vi "Initialisieren.vi"(5 "YAchsen%Max":dbl=1.2, 6 "MFC Cluster Array":refnum<vi>[](array[refnum]), 7 "TestKonfig (Eingang)":T1 {"TestKonfig Interferent"."Gasflasche MFC3" items=["----"=10000, "IAG NH3 3000"=0, "IAG NH3 200"=1, "IAG NH3 2000"=2, "IAG MG"=3, "IAG O2"=4]; "TestKonfig Interferent"."Gasflasche MFC2" items=["----"=10000, "IAG NH3 3000"=0, "IAG NH3 200"=1, "IAG NH3 2000"=2, "IAG MG"=3, "IAG O2"=4]; "TestKonfig Interferent"."Eingangs Konzentration MFC1" min=0.0; "TestKonfig Interferent"."Ausgangs Konzentration MFC1" min=0.0; "TestKonfig Interferent"."MFC2" items=["MFC 2", "MFC 3", "MFC 4", "MFC 5"]; "TestKonfig Interferent"."MFC3" items=["MFC 2", "MFC 3", "MFC 4", "MFC 5"]; "TestKonfig Interferent"."Ausgangs Konzentration MFC3" min=0.0; "TestKonfig Interferent"."Eingangs Konzentration MFC3" min=0.0; "TestKonfig Interferent"."Ausgangs Konzentration MFC2" min=0.0; "TestKonfig Interferent"."Eingangs Konzentration MFC2" min=0.0; "TestKonfig H2O"."HovaCAL Temperature" format="%.2f"; "TestKonfig H2O"."HovaCAL Flow Input Cluster"."HovaCAL Flow Input Cluster" format="%.2f"; "TestKonfig H2O"."Eingangs Konzentration:" min=0.0; "TestKonfig H2O"."zusätzliche Zeitdauer Erster Punkt" min=30 step=1 format="%#_5g"; "TestKonfig H2O"."Zeitdauer Stufen" format="%#_5g"; "TestKonfig H2O"."Max Fehler" format="%#_5g"; "TestKonfig H2O"."Anzahl Stufen" format="%#_5g"; "TestKonfig H2O"."Modus" items=["Messen", "CG zu Entnahmestelle"]}, 8 "Fehler (Eingang)":errorcluster, 9 "Strings Array in":refnum<vi>[](array[refnum]), 10 "Ergebnis  Array in":refnum<vi>[](array[refnum]), 11 "Signalverlaufsdiagramm (Eingang)":refnum<vi>[](array[refnum])) -> (0 "Fehler (Ausgang)":errorcluster, 1 "Strings Array out":refnum<vi>[](array[refnum]), 2 "Ergenis Arry out":refnum<vi>[](array[refnum]), 3 "Signalverlaufsdiagramm (Ausgang)":refnum<vi>[](array[refnum]))   [LabVIEW 2020, in "EPA 1065.lvlib" / "HovaCAL Interference verificaton.lvlib"]
uses:
  HovaCAL Interference verificaton.lvlib
  TestKonfig.ctl
  TestKonfig H2O.ctl
  Modus.ctl
  Linearisierung V2/SpanEinstellungen/Einheit.ctl
  Linearisierung V2/Gasteiler/Stufen Tabelle 10 Stufen.ctl
  Linearisierung V2/Gasteiler/HovaCAL_Interface/Controls/Flow Einstellung.ctl
  Linearisierung V2/Gasteiler/HovaCAL_Interface/Controls/Temp Sollwerte Anzeige.ctl
  TestKonfig Interferents.ctl
  MFCAuswahl.ctl
  Seiten/System Einstellungen V2/Gasflasche Auswahl.ctl
  Linearisierung V2/SpanEinstellungen/SpanEinstellungen.lvlib
  Linearisierung V2/Gasteiler/HovaCAL_Interface/Controls/Controls.lvlib
  Seiten/System Einstellungen V2/System Einstellungen V2.lvlib
  Linearisierung V2/Gasteiler/Gasteiler.lvlib
panel:
  # "sec"
  # "%"
  # "sec"
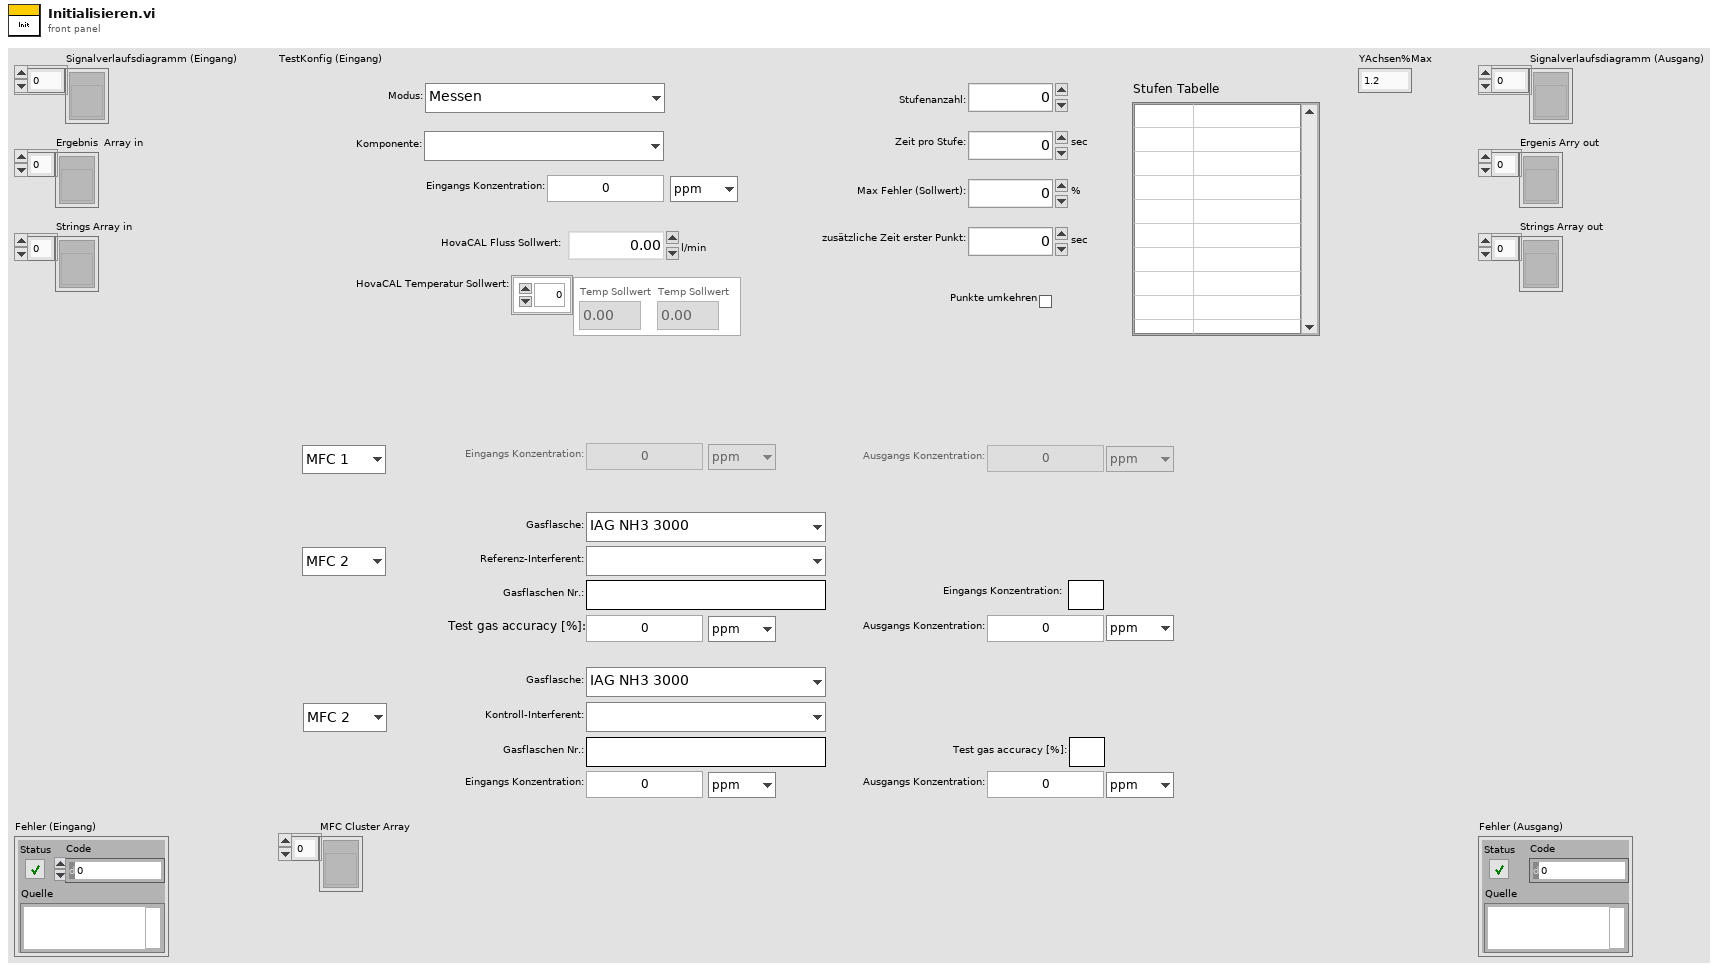
[diagram p1: front panel]
types:
  T1 = typedef "EPA 1065.lvlib/HovaCAL Interference verificaton.lvlib/TestKonfig.ctl" = cluster{"TestKonfig H2O":T2, "TestKonfig Interferent":T8}
  T2 = typedef "EPA 1065.lvlib/HovaCAL Interference verificaton.lvlib/TestKonfig H2O.ctl" = cluster{"Modus":T3, "Komponente:":u16, "Eingangs Konzentration:":dbl, "Einheit":T4, "Anzahl Stufen":sgl, "Zeitdauer Stufen":sgl, "Max Fehler":sgl, "zusätzliche Zeitdauer Erster Punkt":sgl, "Punkte umkehren":bool, "Stufen Tabelle":T5, "HovaCAL Flow Input Cluster":T6, "HovaCAL Temperature":T7}
  T3 = typedef "EPA 1065.lvlib/HovaCAL Interference verificaton.lvlib/Modus.ctl" = u16
  T4 = typedef "Linearisierung v2.lvlib/SpanEinstellungen.lvlib/Einheit.ctl" = enum16{"ppm", "%"}
  T5 = typedef "Linearisierung v2.lvlib/Gasteiler.lvlib/Stufen Tabelle 10 Stufen.ctl" = string[][]
  T6 = typedef "Linearisierung v2.lvlib/Gasteiler.lvlib/HovaCAL_Interface.lvlib/Controls.lvlib/Flow Einstellung.ctl" = cluster{"HovaCAL Flow Input Cluster":dbl}
  T7 = typedef "Linearisierung v2.lvlib/Gasteiler.lvlib/HovaCAL_Interface.lvlib/Controls.lvlib/Temp Sollwerte Anzeige.ctl" = dbl[]
  T8 = typedef "EPA 1065.lvlib/HovaCAL Interference verificaton.lvlib/TestKonfig Interferents.ctl" = cluster{"MFC1":enum16{"MFC 1"}, "Eingangs Konzentration MFC1":dbl, "Einheit MFC1 Eingang":T4, "Ausgangs Konzentration MFC1":dbl, "Einheit MFC1 Ausgang":T4, "MFC2":T9, "Referenz-Interferent:":u16, "Gasflaschen Nr MFC2":string, "Accuracy MFC2":string, "Eingangs Konzentration MFC2":dbl, "Einheit MFC2 Eingang":T4, "Ausgangs Konzentration MFC2":dbl, "Einheit MFC2 Ausgang":T4, "MFC3":T9, "Kontroll-Interferent:":u16, "Gasflaschen Nr MFC3":string, "Accuracy MFC3":string, "Eingangs Konzentration MFC3":dbl, "Einheit MFC3 Eingang":T4, "Ausgangs Konzentration MFC3":dbl, "Einheit MFC3 Ausgang":T4, "Gasflasche MFC2":T10, "Gasflasche MFC3":T10}
  T9 = typedef "EPA 1065.lvlib/HovaCAL Interference verificaton.lvlib/MFCAuswahl.ctl" = u16
  T10 = typedef "System Einstellungen V2.lvlib/Gasflasche Auswahl.ctl" = u16
  T11 = enum8{"Enabled", "Disabled", "Disabled and Grayed Out"}
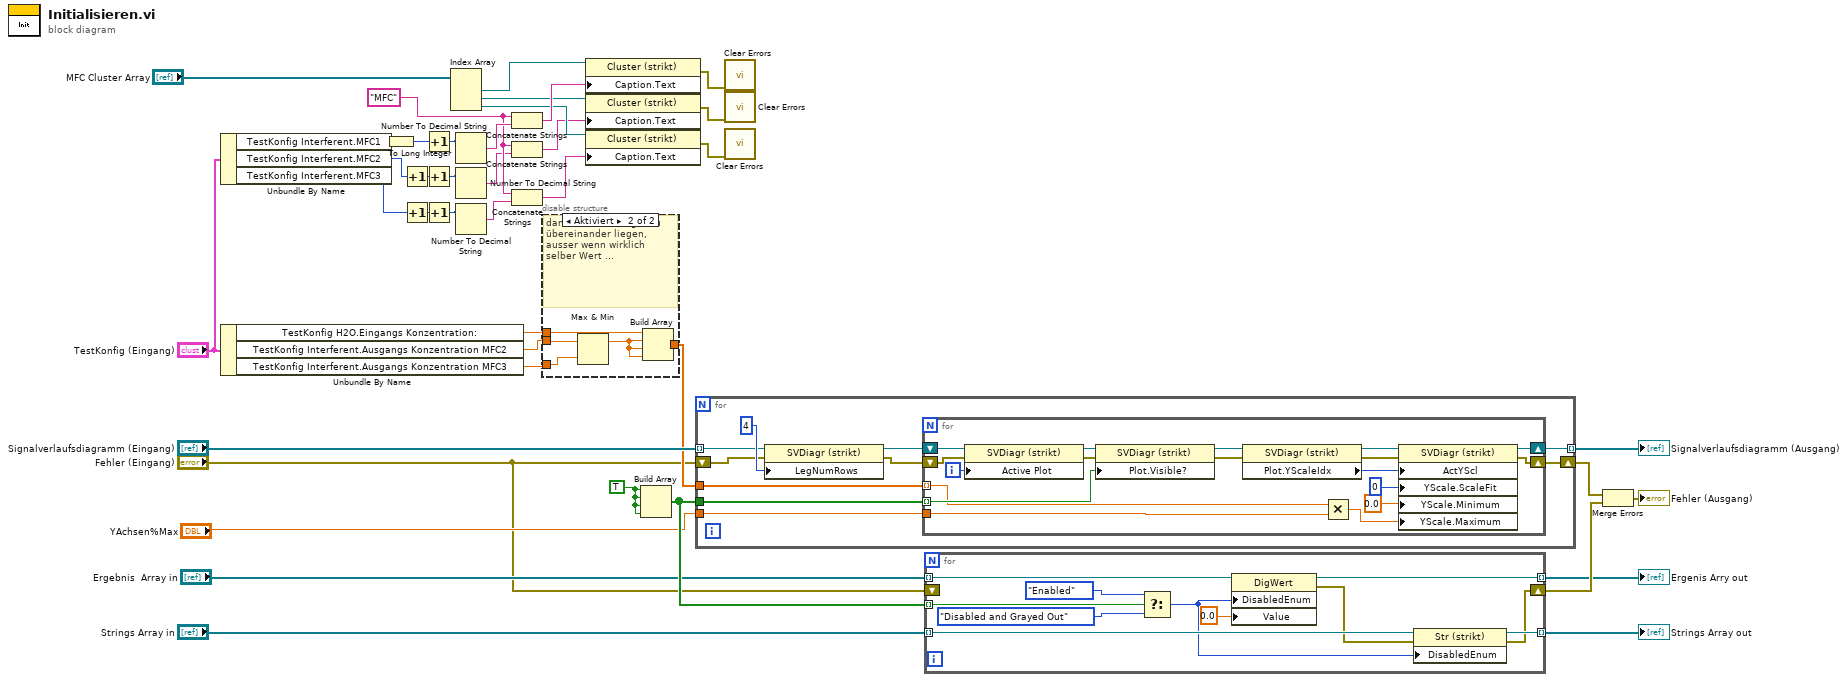
[diagram p0: block diagram]
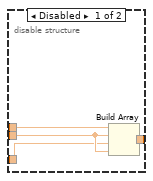
[diagram p2: hidden frame]
diagram:
  w7 = "MFC"
  w31 = TRUE
  n1 = Unbundle By Name("TestKonfig (Eingang)") -> ("TestKonfig Interferent.MFC1"=w22:enum16{"MFC 1"}, "TestKonfig Interferent.MFC2"=w11:T9, "TestKonfig Interferent.MFC3"=w9:T9)
  n2 = Unbundle By Name("TestKonfig (Eingang)") -> ("TestKonfig H2O.Eingangs Konzentration:"=w30:dbl, "TestKonfig Interferent.Ausgangs Konzentration MFC2"=w26:dbl, "TestKonfig Interferent.Ausgangs Konzentration MFC3"=w25:dbl)
  n3 = To Long Integer(number=w22) -> (32bit integer=w2:i32)
  n4 = Increment(x=w11) -> (x+1=w10:T9)
  n5 = Increment(x=w9) -> (x+1=w8:T9)
  n6 = Increment(x=w2) -> (x+1=w20:i32)
  n7 = Increment(x=w10) -> (x+1=w13:T9)
  n8 = Increment(x=w8) -> (x+1=w12:T9)
  n9 = Index Array(array="MFC Cluster Array") -> (element #1=w23:refnum<vi>, element #2=w18:refnum<vi>, element #3=w17:refnum<vi>)  [unwired: 3 in]
  n10 = Number To Decimal String(number=w20) -> (decimal integer string=w21:string)  [unwired: 1 in]
  n11 = Number To Decimal String(number=w13) -> (decimal integer string=w6:string)  [unwired: 1 in]
  n12 = Number To Decimal String(number=w12) -> (decimal integer string=w5:string)  [unwired: 1 in]
  n13 = Concatenate Strings(w7, w21) -> (w19:string)
  n14 = Concatenate Strings(w7, w6) -> (w4:string)
  n15 = Concatenate Strings(w7, w5) -> (w3:string)
  n16 = disable-structure shown="Aktiviert" {
    disable-tunnel: w30 -> [w45 w50]
    disable-tunnel: [w44 w49] -> w29
    disable-tunnel: w26 -> [w43 w48]
    disable-tunnel: w25 -> [w42 w47]
    frame Disabled {
      n17 = Build Array(w45, w43, w42, w43) -> (w44:dbl[])
    }
    frame Enabled {
      # "damit Kurven nie genau übereinander liegen, ausser wenn wirklich selber Wert ..."
      n18 = Max & Min(x=w48, y=w47) -> (max(x,y)=w46:dbl)  [unwired: 1 out]
      n19 = Build Array(w50, w46, w46, w46) -> (w49:dbl[])
    }
  }
  n20 = property class="Cluster (strikt)"(reference=w23, "Caption.Text"=w19) -> (error out=w16:errorcluster)  [unwired: 1 in, 1 out]
  n21 = property class="Cluster (strikt)"(reference=w18, "Caption.Text"=w4) -> (error out=w15:errorcluster)  [unwired: 1 in, 1 out]
  n22 = property class="Cluster (strikt)"(reference=w17, "Caption.Text"=w3) -> (error out=w14:errorcluster)  [unwired: 1 in, 1 out]
  n23 = Build Array(w31, w31, w31, w31) -> (w40:bool[])
  n24 = for {
    tunnel: w40 -> [w60]
    tunnel: "Signalverlaufsdiagramm (Eingang)" -> [w56] mode=indexing
    tunnel: [w58] -> w34 mode=indexing
    shift-right: [w59] -> w36
    shift-left: "Fehler (Eingang)" -> [w54]
    tunnel: w29 -> [w52]
    tunnel: "YAchsen%Max" -> [w51]
    n25 = property class="SVDiagr (strikt)"(reference=w56, error in=w54, "LegNumRows"=u32 4 ("Legende:Zeilenanzahl")) -> (reference out=w55:refnum<vi>, error out=w53:errorcluster)
    n26 = for {
      shift-right: [w75] -> w59
      shift-left: w53 -> [w74]
      tunnel: w60 -> [w73] mode=indexing
      shift-right: [w68] -> w58
      shift-left: w55 -> [w72]
      tunnel: w52 -> [w66] mode=indexing
      tunnel: w51 -> [w64]
      i -> [w67]
      n27 = property on="Eigenschaftsknoten" class="SVDiagr (strikt)"(reference=w72, error in=w74, "Active Plot"=w67) -> (reference out=w71:refnum<vi>, error out=w76:errorcluster)
      n28 = property on="Eigenschaftsknoten" class="SVDiagr (strikt)"(reference=w71, error in=w76, "Plot.Visible?"=w73) -> (reference out=w70:refnum<vi>, error out=w77:errorcluster)
      n29 = property on="Eigenschaftsknoten" class="SVDiagr (strikt)"(reference=w70, error in=w77) -> (reference out=w69:refnum<vi>, error out=w78:errorcluster, "Plot.YScaleIdx"=w62:u32)
      n30 = Multiply(x=w66, y=w64) -> (x*y=w65:dbl)
      n31 = property on="Eigenschaftsknoten" class="SVDiagr (strikt)"(reference=w69, error in=w78, "ActYScl"=w62, "YScale.ScaleFit"=u8 0 ("Y-Achse.Achsenanpassung"), "YScale.Minimum"=0.0 ("Y-Achse.Bereich:Minimum"), "YScale.Maximum"=w65) -> (reference out=w68:refnum<vi>, error out=w75:errorcluster)
    }
  }
  "Signalverlaufsdiagramm (Ausgang)" <- w34
  n32 = call <vilib>:"Clear Errors.vi"("error in (no error)"=w16) -> ()  [unwired: 5 in, 2 out]
  n33 = call <vilib>:"Clear Errors.vi"("error in (no error)"=w15) -> ()  [unwired: 5 in, 2 out]
  n34 = call <vilib>:"Clear Errors.vi"("error in (no error)"=w14) -> ()  [unwired: 5 in, 2 out]
  n35 = for {
    tunnel: w40 -> [w84] mode=indexing
    tunnel: "Ergebnis  Array in" -> [w89] mode=indexing
    tunnel: "Strings Array in" -> [w88] mode=indexing
    tunnel: [w83] -> w33 mode=indexing
    tunnel: [w82] -> w32 mode=indexing
    shift-right: [w80] -> w41
    shift-left: "Fehler (Eingang)" -> [_]
    n36 = Select(t=T11."Enabled" ("Deaktiviert"), s=w84, f=T11."Disabled and Grayed Out" ("Deaktiviert")) -> (s? t:f=w85:T11)
    n37 = property class="DigWert"(reference=w89, "DisabledEnum"=w85, "Value"=0.0 ("Y-Achse.Bereich:Minimum")) -> (reference out=w83:refnum<vi>, error out=w81:errorcluster)  [unwired: 1 in]
    n38 = property class="Str (strikt)"(reference=w88, error in=w81, "DisabledEnum"=w85) -> (reference out=w82:refnum<vi>, error out=w80:errorcluster)
  }
  "Ergenis Arry out" <- w33
  "Strings Array out" <- w32
  n39 = Merge Errors(w36, w41) -> (→"Fehler (Ausgang)":errorcluster)
